vi "Process Command.vi"(4 "error in (no error)":errorcluster, 7 "Set Acquisition Rate in":refnum<class "Remote Access Commands_Set Acquisition Rate.lvclass">) -> (0 "error out":errorcluster, 2 "Response out":T1, 3 "Set Acquisition Rate out":refnum<class "Remote Access Commands_Set Acquisition Rate.lvclass">)   [LabVIEW 2020, in "Startup Processes.lvlib" / "Remote Access Commands_Set Acquisition Rate.lvclass"]
uses:
  Remote Access Commands_Set Acquisition Rate.lvclass
  Remote Access Commands_Set Acquisition Rate.lvclass/Remote Access Commands_Set Acquisition Rate.ctl
  toolbox/Standard Signalling/not_Generic Named Notifier/not_Generic Named Notifier.lvlib
  Remote Access Commands.lvclass
  Startup Processes.lvlib
  _typedefs/Custom Remote Access Error Codes.ctl
  _ude/Set Acquisition Rate/Set Acquisition Rate.lvlib
  C:/Users/Fred Guo/Desktop/Release 19/_libraries/Startup Processes/_classes/Remote Access Commands/Remote Access Commands.lvclass
  C:/Users/Fred Guo/Desktop/Release 19/_libraries/Startup Processes/_classes/Remote Access Commands/Set Acquisition Rate/Remote Access Commands_Set Acquisition Rate.lvclass
  _typedefs/JSON Response Cluster.ctl
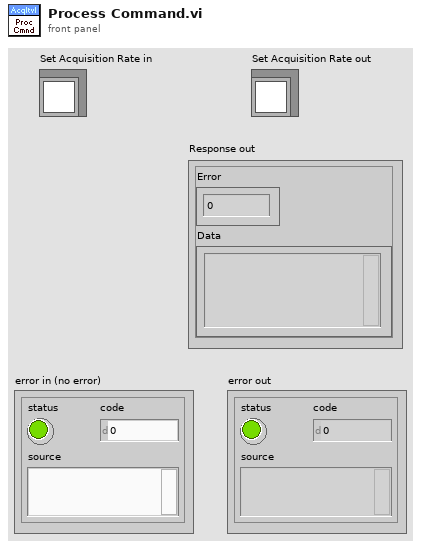
[diagram p1: front panel]
types:
  T1 = typedef "Startup Processes.lvlib/JSON Response Cluster.ctl" = cluster{"Error":i32, "Data":string}
  T2 = typedef "Startup Processes.lvlib/Custom Remote Access Error Codes.ctl" = enum16{"No Error", "CRC Error", "Update Failed"}
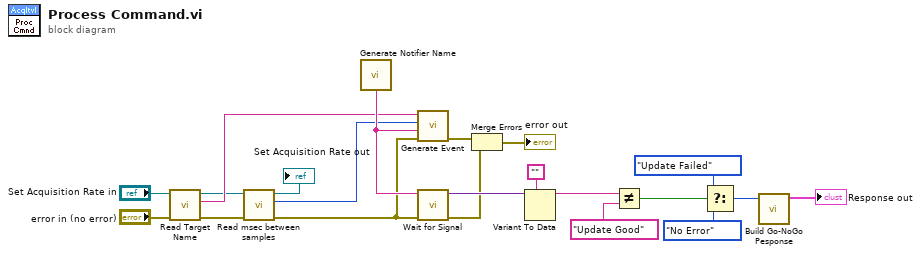
[diagram p0: block diagram]
diagram:
  n1 = call "Read Target Name.vi"("Error In"="error in (no error)", "Remote Access Commands in"="Set Acquisition Rate in") -> ("Error Out"=w9:errorcluster, "Target Name"=w16:string, "Remote Access Commands out"=w11:refnum<class "Remote Access Commands_Set Acquisition Rate.lvclass">)  [unwired: 3 in]
  n2 = call-dynamic "Read msec between samples.vi"("Error In"=w9, "Set Acquisition Rate in"=w11) -> ("Error Out"=w8:errorcluster, "msec between samples"=w7:i32, "Set Acquisition Rate out"=→"Set Acquisition Rate out":refnum<class "Remote Access Commands_Set Acquisition Rate.lvclass">)  [unwired: 3 in]
  n3 = call "Generate Notifier Name.vi"() -> ("Notifier Name"=w20:string)
  n4 = call "Generate Event.vi"("Error In"=w8, "Response Notifier"=w20, "Sample Period"=w7, "Source Name"=w16) -> ("Error Out"=w21:errorcluster)  [unwired: 3 in]
  n5 = call "Wait for Signal.vi"("Error In"=w8, "Notifier Name"=w20) -> ("Error Out"=w12:errorcluster, "Signal Data"=w15:variant)  [unwired: 4 in]
  n6 = Merge Errors(w21, w12) -> (→"error out":errorcluster)
  n7 = Variant To Data(type="", Variant=w15) -> (data=w3:string)  [unwired: 1 in, 1 out]
  n8 = Not Equal?(x=w3, y="Update Good") -> (x != y?=w2:bool)
  n9 = Select(t=Custom_Remote_Access_Error_Codes."Update Failed" ("Error"), s=w2, f=Custom_Remote_Access_Error_Codes."No Error" ("Error")) -> (s? t:f=w4:T2)
  n10 = call "Build Go-NoGo Pesponse.vi"("Error"=w4) -> ("Response"=→"Response out":T1)  [unwired: 5 in, 1 out]
